vi "XYMOVEMENTEW.vi"() -> ()   [LabVIEW 2021]
panel:
  out "Obstacle Control":i32
  in  "Facing XY x=0 y=1 in":i32
  in  "x move":i32
  in  "Y move":i32
  out "Facing XY x=0 y=1 out":i32
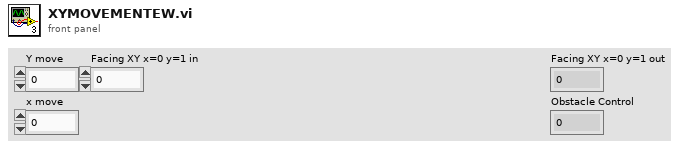
[diagram p1: front panel]
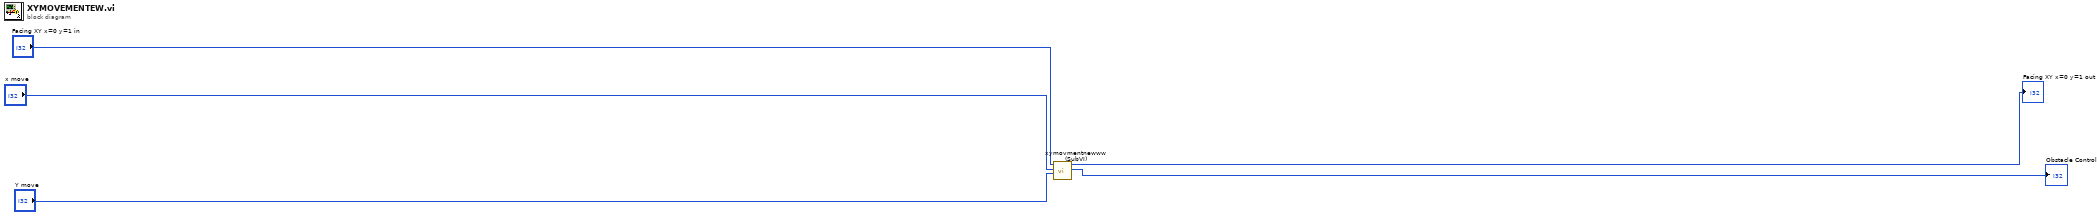
[diagram p0: block diagram]
diagram:
  n1 = call "xymovmentnewww (SubVI).vi"("Y move"="Y move", "x move"="x move", "Facing XY x=0 y=1 in"="Facing XY x=0 y=1 in") -> ("Obstacle Condition"=→"Obstacle Control":i32, "Facing XY x=0 y=1 out"=→"Facing XY x=0 y=1 out":i32)  [unwired: 7 in]
